vi "ForecastData Test.vi"(8 "error in":errorcluster, 11 "IED Test in":refnum<class "IED Test.lvclass">) -> (0 "error out":errorcluster, 2 "Test Result":T1=enum."Success", 3 "IED Test out":refnum<class "IED Test.lvclass">)   [LabVIEW 2018, in "IED Test Framework.lvlib" / "IED Test.lvclass"]
uses:
  IED Test.lvclass
  C:/Program Files (x86)/National Instruments/LabVIEW 2018/vi.lib/ActorFramework/Actor/Actor.lvclass
  C:/Users/Administrator/Desktop/2018LabVIEW EMS/EMS Generic Actor/EMS Generic/EMS Generic.lvclass
  Controls/Test Result.ctl
  <vilib>/ORNL/CSEISMIC DDS/CSEISMIC DDS Base/Data Types/Controls/DeviceClass Selector.ctl
  ForecastData Actor/ForecastData/ForecastData.lvclass
  C:/Users/Administrator/Desktop/2018LabVIEW EMS/IED Actors/Device DDS Communications Framework/Device DDS Communications/Device DDS Communications.lvclass
  <vilib>/ORNL/CSEISMIC DDS/CSEISMIC DDS Base/CSEISMIC DDS.lvclass/CSEISMIC DDS.ctl
  <vilib>/ORNL/CSEISMIC DDS/CSEISMIC DDS Base/Data Types/Controls/DeviceID.ctl
  <vilib>/ActorFramework/Message Enqueuer/Message Enqueuer.lvclass/Message Enqueuer.ctl
  <vilib>/ORNL/CSEISMIC DDS/CSEISMIC DDS Base/Accessors/Write DDS Reference.vi
  <vilib>/ORNL/CSEISMIC DDS/CSEISMIC DDS Base/Accessors/Read DDS Reference.vi
  <vilib>/ActorFramework/Message Enqueuer/Enqueue.vi
  <vilib>/ORNL/CSEISMIC DDS/DDS Writer/DDS Writer.lvclass
  C:/Program Files (x86)/National Instruments/LabVIEW 2018/vi.lib/ORNL/CSEISMIC DDS/CSEISMIC DDS Base/CSEISMIC DDS.lvclass
  <vilib>/ActorFramework/Stop Msg/Stop Msg.lvclass
  C:/Program Files (x86)/National Instruments/LabVIEW 2018/vi.lib/ActorFramework/Message/Message.lvclass
  <vilib>/ORNL/CSEISMIC DDS/CSEISMIC DDS Base/Error Handler.vi
  <vilib>/ActorFramework/Message Priority Queue/Priority Enqueue.vi
  <vilib>/ORNL/CSEISMIC DDS/CSEISMIC DDS Base/CSEISMIC DDS.lvclass
  Device DDS Communications Framework/Device DDS Communications/Device DDS Communications.lvclass
  <vilib>/ActorFramework/Actor/Actor.lvclass
  EMS Generic Actor/EMS Generic/EMS Generic.lvclass
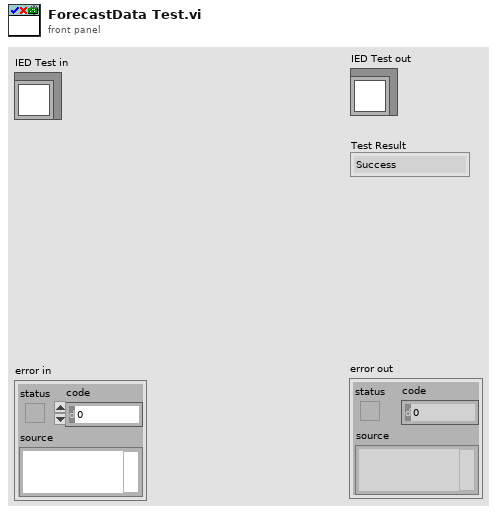
[diagram p1: front panel]
types:
  T1 = typedef "IED Test Framework.lvlib/IED Test.lvclass/Test Result.ctl" = enum16{"Invalid", "Success", "Failure", "Error", "Timeout"}
  T2 = typedef "CSEISMIC DDS.lvlib/CSEISMIC DDS.lvclass/DeviceID.ctl" = string
  T3 = typedef "CSEISMIC DDS.lvlib/CSEISMIC DDS.lvclass/DeviceClass Selector.ctl" = u16
  T4 = typedef "CSEISMIC DDS.lvlib/CSEISMIC DDS.lvclass/ForecastData_Data.ctl" = cluster{"DeviceID":T2, "TargetID":T2, "t0":dbl, "dt":dbl, "Magnitude":dbl[]}
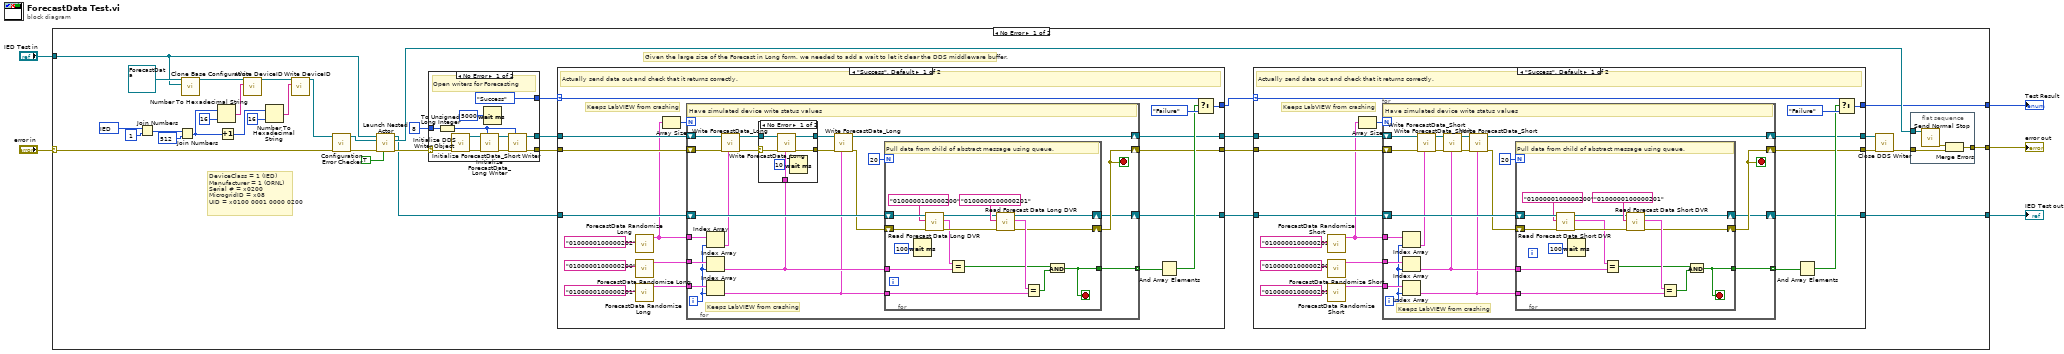
[diagram p0: block diagram]
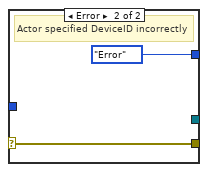
[diagram p5: hidden frame]
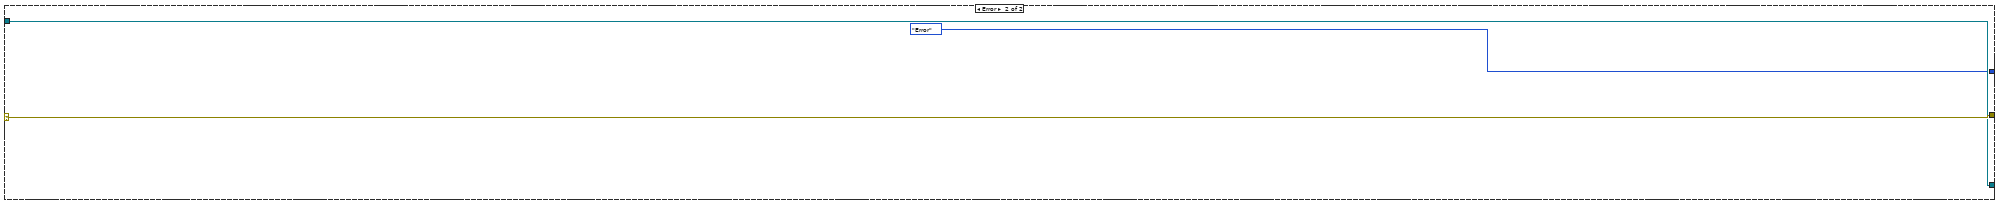
[diagram p6: hidden frame]
diagram:
  n1 = case shown="No Error" "error in" {
    selector: "error in" -> [w37 w185]
    tunnel: [w39 w185] -> w2
    tunnel: [w6 w184] -> w1
    tunnel: "IED Test in" -> [w8 w184]
    tunnel: [w12 Test_Result."Error" ("f")] -> w3
    frame No Error {
      w30 = T3 256 items=["Invalid"=0, "IED"=256, "DER"=512, "Relay"=768, "Meter"=1024, "Load"=1280, "Forecast"=1536, "Price"=1792, "Energy Storage"=513, "PV"=514, "Generator"=515, "Smart Relay"=769, "PCC"=770, "Smart Meter"=1025, "PMU"=1026, "HVAC"=1281] ("DeviceClass")
      # "Given the large size of the Forecast in Long form, we needed to add a wait to let it clear the DDS middleware buffer."
      # "DeviceClass = 1 (IED)\nManufacturer = 1 (ORNL)\nSerial # = x0200\nMicrogridID = x08\nUID = x0100 0001 0000 0200"
      n2 = Join Numbers(hi=w30, lo=u16 1 ("MicrogridID")) -> ((hi.lo)=w27:u32)
      n3 = Join Numbers(hi=w27, lo=u32 512 ("MicrogridID")) -> ((hi.lo)=w32:u64)
      n4 = call-dynamic "Clone Base Configuration.vi"("Source Object"=w8, "Target Object in"=refnum<class "ForecastData.lvclass"> refnum ("ForecastData Actor.lvlib:ForecastData.lvclass")) -> ("Target Object out"=w9:refnum<class "ForecastData.lvclass">)  [unwired: 9 in]
      n5 = Number To Hexadecimal String(1:i16 16 ("width (-)"), 2:w32) -> (0:w25:string)
      n6 = Increment(x=w32) -> (x+1=w34:u64)
      n7 = call-dynamic "Write DeviceID.vi"("DeviceID"=w25, "Device DDS Communications in"=w9) -> ("Device DDS Communications out"=w29:refnum<class "ForecastData.lvclass">)  [unwired: 9 in]
      n8 = Number To Hexadecimal String(1:i16 16 ("width (-)"), 2:w34) -> (0:w35:string)
      n9 = call-dynamic "Write DeviceID.vi"("DeviceID"=w35, "Device DDS Communications in"=w29) -> ("Device DDS Communications out"=w11:refnum<class "ForecastData.lvclass">)  [unwired: 9 in]
      n10 = call "Configuration Error Checker.vi"("error in"=w37, "Device DDS Communications in"=w11) -> ("error out"=w40:errorcluster, "Device DDS Communications out"=w38:refnum<class "ForecastData.lvclass">)  [unwired: 8 in]
      n11 = call <vilib>:"Launch Nested Actor.vi"("Open Actor Core front panel? (F)"=TRUE, "error in (no error)"=w40, "Nested Actor"=w38, "Caller Actor in"=w8) -> ("error out"=w23:errorcluster, "Nested Actor's Enqueuer"=w36:refnum<class "Message Enqueuer.lvclass">, "Caller Actor out"=w16:refnum<class "IED Test.lvclass">)  [unwired: 5 in]
      n12 = case shown="No Error" w23 {
        selector: w23 -> [w178 w182]
        tunnel: [w171 w182] -> w20
        tunnel: u32 8 ("domain id") -> [w180 _]
        tunnel: [Test_Result."Success" ("Test Result in") Test_Result."Error" ("Test Result")] -> w22
        tunnel: [w170 _] -> w21
        frame No Error {
          # "Open writers for Forecasting"
          n13 = To Unsigned Long Integer(number=w180) -> (unsigned 32bit integer=w173:u32)
          n14 = call <vilib>:"Initialize DDS Writer Object.vi"("error in"=w178) -> ("error out"=w177:errorcluster, "DDS Writer out"=w176:refnum<class "DDS Writer.lvclass">)  [unwired: 9 in]
          n15 = call <vilib>:"Initialize ForecastData_Long Writer.vi"("MicrogridID"=w173, "error in"=w177, "DDS Writer in"=w176) -> ("error out"=w174:errorcluster, "DDS Writer out"=w175:refnum<class "DDS Writer.lvclass">)  [unwired: 7 in]
          n16 = Wait (ms)(milliseconds to wait=u32 5000) -> ()  [unwired: 1 out]
          n17 = call <vilib>:"Initialize ForecastData_Short Writer.vi"("MicrogridID"=w173, "error in"=w174, "DDS Writer in"=w175) -> ("error out"=w171:errorcluster, "DDS Writer out"=w170:refnum<class "DDS Writer.lvclass">)  [unwired: 7 in]
        }
        frame Error {
          # "Actor specified DeviceID incorrectly"
        }
      }
      n18 = case shown="\"Success\", Default" w22 {
        selector: w22 -> [w120 w168]
        tunnel: w21 -> [w121 w167]
        tunnel: w16 -> [w115 w166]
        tunnel: w20 -> [w116 w169]
        tunnel: [w118 w168] -> w17
        tunnel: [w114 w169] -> w18
        tunnel: [w112 w167] -> w19
        tunnel: [w104 w166] -> w7
        frame "Success", Default {
          # "Keeps LabVIEW from crashing"
          # "Actually send data out and check that it returns correctly."
          n19 = call "ForecastData Randomize Long.vi"("DeviceID"=T2 "0100000100000202" ("(hi.lo)")) -> ("ForecastData_Long Array out"=w111:T4[])  [unwired: 10 in]
          n20 = call "ForecastData Randomize Long.vi"("DeviceID"=T2 "0100000100000200" ("(hi.lo)")) -> ("ForecastData_Long Array out"=w106:T4[])  [unwired: 10 in]
          n21 = call "ForecastData Randomize Long.vi"("DeviceID"=T2 "0100000100000201" ("(hi.lo)")) -> ("ForecastData_Long Array out"=w107:T4[])  [unwired: 10 in]
          n22 = Array Size(array=w111) -> (size(s)=w113:i32)
          n23 = for {
            N: w113 -> [_]
            shift-right: [w138] -> w112
            shift-left: w121 -> [w141]
            tunnel: w111 -> [w134]
            tunnel: w107 -> [w129]
            tunnel: w106 -> [w130]
            shift-right: [w131] -> w114
            shift-left: w116 -> [w137]
            shift-right: [w125] -> w104
            shift-left: w115 -> [w133]
            tunnel: [w122] -> w105 mode=indexing
            i -> [w127]
            stop <- w131 stop-if-true
            # "Keeps LabVIEW from crashing"
            # "Have simulated device write status values"
            n24 = Index Array(array=w134, index=w127) -> (element=w126:T4)
            n25 = Index Array(array=w130, index=w127) -> (element=w124:T4)
            n26 = Index Array(array=w129, index=w127) -> (element=w123:T4)
            n27 = call <vilib>:"Write ForecastData_Long.vi"("ForecastData"=w126, "error in"=w137, "DDS Writer in"=w141) -> ("error out"=w136:errorcluster, "DDS Writer out"=w140:refnum<class "DDS Writer.lvclass">)  [unwired: 7 in]
            n28 = case shown="No Error" w136 {
              selector: w136 -> [w145 w148]
              tunnel: w140 -> [w147 w149]
              tunnel: [w146 w149] -> w139
              tunnel: [w144 w148] -> w135
              tunnel: w124 -> [w143 _]
              frame No Error {
                n29 = call <vilib>:"Write ForecastData_Long.vi"("ForecastData"=w143, "error in"=w145, "DDS Writer in"=w147) -> ("error out"=w144:errorcluster, "DDS Writer out"=w146:refnum<class "DDS Writer.lvclass">)  [unwired: 7 in]
                n30 = Wait (ms)(milliseconds to wait=u32 10) -> ()  [unwired: 1 out]
              }
              frame Error {
              }
            }
            n31 = call <vilib>:"Write ForecastData_Long.vi"("ForecastData"=w123, "error in"=w135, "DDS Writer in"=w139) -> ("error out"=w132:errorcluster, "DDS Writer out"=w138:refnum<class "DDS Writer.lvclass">)  [unwired: 7 in]
            n32 = for {
              N: 20 -> [_]
              shift-right: [w154] -> w131
              shift-left: w132 -> [w164]
              shift-right: [w155] -> w125
              shift-left: w133 -> [w165]
              tunnel: w124 -> [w159]
              tunnel: w123 -> [w157]
              tunnel: [w151] -> w122
              stop <- w151 stop-if-true
              # "Pull data from child of abstract message using queue."
              n33 = Wait (ms)(milliseconds to wait=u32 100) -> ()  [unwired: 1 out]
              n34 = call "Read Forecast Data Long DVR.vi"("error in"=w164, "DeviceID"=T2 "0100000100000200" ("(hi.lo)"), "EMS Generic in"=w165) -> ("error out"=w160:errorcluster, "ForecastData"=w158:T4, "EMS Generic out"=w161:refnum<class "IED Test.lvclass">)  [unwired: 5 in, 1 out]
              n35 = Equal?(x=w158, y=w159) -> (x = y?=w153:bool)
              n36 = call "Read Forecast Data Long DVR.vi"("error in"=w160, "DeviceID"=T2 "0100000100000201" ("(hi.lo)"), "EMS Generic in"=w161) -> ("error out"=w154:errorcluster, "ForecastData"=w156:T4, "EMS Generic out"=w155:refnum<class "IED Test.lvclass">)  [unwired: 5 in, 1 out]
              n37 = Equal?(x=w156, y=w157) -> (x = y?=w152:bool)
              n38 = And(x=w153, y=w152) -> (x .and. y?=w151:bool)
            }
          }
          n39 = And Array Elements(Boolean array=w105) -> (logical AND=w117:bool)
          n40 = Select(t=w120, s=w117, f=Test_Result."Failure") -> (s? t:f=w118:T1)
        }
        frame "Error" {
        }
      }
      n41 = case shown="\"Success\", Default" w17 {
        selector: w17 -> [w62 w102]
        tunnel: w19 -> [w63 w101]
        tunnel: w7 -> [w57 w100]
        tunnel: w18 -> [w58 w103]
        tunnel: [w60 w102] -> w12
        tunnel: [w56 w103] -> w14
        tunnel: [w54 w101] -> w15
        tunnel: [w47 w100] -> w6
        frame "Success", Default {
          # "Keeps LabVIEW from crashing"
          # "Actually send data out and check that it returns correctly."
          n42 = call "ForecastData Randomize Short.vi"("DeviceID"=T2 "0100000100000202" ("(hi.lo)")) -> ("ForecastData_Short Array out"=w53:T4[])  [unwired: 10 in]
          n43 = call "ForecastData Randomize Short.vi"("DeviceID"=T2 "0100000100000200" ("(hi.lo)")) -> ("ForecastData_Short Array out"=w48:T4[])  [unwired: 10 in]
          n44 = call "ForecastData Randomize Short.vi"("DeviceID"=T2 "0100000100000201" ("(hi.lo)")) -> ("ForecastData_Short Array out"=w49:T4[])  [unwired: 10 in]
          n45 = Array Size(array=w53) -> (size(s)=w55:i32)
          n46 = for {
            N: w55 -> [_]
            shift-right: [w80] -> w54
            shift-left: w63 -> [w83]
            tunnel: w53 -> [w76]
            tunnel: w49 -> [w71]
            tunnel: w48 -> [w72]
            shift-right: [w73] -> w56
            shift-left: w58 -> [w79]
            shift-right: [w67] -> w47
            shift-left: w57 -> [w75]
            tunnel: [w64] -> w46 mode=indexing
            i -> [w69]
            stop <- w73 stop-if-true
            # "Keeps LabVIEW from crashing"
            # "Have simulated device write status values"
            n47 = Index Array(array=w76, index=w69) -> (element=w68:T4)
            n48 = Index Array(array=w72, index=w69) -> (element=w66:T4)
            n49 = Index Array(array=w71, index=w69) -> (element=w65:T4)
            n50 = call <vilib>:"Write ForecastData_Short.vi"("ForecastData"=w68, "error in"=w79, "DDS Writer in"=w83) -> ("error out"=w78:errorcluster, "DDS Writer out"=w82:refnum<class "DDS Writer.lvclass">)  [unwired: 7 in]
            n51 = call <vilib>:"Write ForecastData_Short.vi"("ForecastData"=w66, "error in"=w78, "DDS Writer in"=w82) -> ("error out"=w77:errorcluster, "DDS Writer out"=w81:refnum<class "DDS Writer.lvclass">)  [unwired: 7 in]
            n52 = call <vilib>:"Write ForecastData_Short.vi"("ForecastData"=w65, "error in"=w77, "DDS Writer in"=w81) -> ("error out"=w74:errorcluster, "DDS Writer out"=w80:refnum<class "DDS Writer.lvclass">)  [unwired: 7 in]
            n53 = for {
              N: 20 -> [_]
              shift-right: [w88] -> w73
              shift-left: w74 -> [w99]
              shift-right: [w87] -> w67
              shift-left: w75 -> [w98]
              tunnel: w66 -> [w92]
              tunnel: w65 -> [w91]
              tunnel: [w84] -> w64
              stop <- w84 stop-if-true
              # "Pull data from child of abstract message using queue."
              n54 = call "Read Forecast Data Short DVR.vi"("error in"=w99, "DeviceID"=T2 "0100000100000200" ("(hi.lo)"), "EMS Generic in"=w98) -> ("error out"=w95:errorcluster, "ForecastData"=w90:T4, "EMS Generic out"=w94:refnum<class "IED Test.lvclass">)  [unwired: 5 in, 1 out]
              n55 = Wait (ms)(milliseconds to wait=u32 100) -> ()  [unwired: 1 out]
              n56 = Equal?(x=w90, y=w92) -> (x = y?=w86:bool)
              n57 = call "Read Forecast Data Short DVR.vi"("error in"=w95, "DeviceID"=T2 "0100000100000201" ("(hi.lo)"), "EMS Generic in"=w94) -> ("error out"=w88:errorcluster, "ForecastData"=w89:T4, "EMS Generic out"=w87:refnum<class "IED Test.lvclass">)  [unwired: 5 in, 1 out]
              n58 = Equal?(x=w89, y=w91) -> (x = y?=w85:bool)
              n59 = And(x=w86, y=w85) -> (x .and. y?=w84:bool)
            }
          }
          n60 = And Array Elements(Boolean array=w46) -> (logical AND=w59:bool)
          n61 = Select(t=w62, s=w59, f=Test_Result."Failure") -> (s? t:f=w60:T1)
        }
        frame "Error" {
        }
      }
      n62 = call <vilib>:"Close DDS Writer.vi"("error in"=w14, "DDS Writer in"=w15) -> ("error out"=w13:errorcluster)  [unwired: 9 in]
      n63 = flat-sequence {
        tunnel: w36 -> [w45]
        tunnel: [w43] -> w39
        tunnel: w13 -> [w42]
        frame #0 {
          n64 = call <vilib>:"Send Normal Stop.vi"("Message Enqueuer"=w45) -> ("error out"=w44:errorcluster)  [unwired: 10 in]
          n65 = Merge Errors(w44, w42) -> (w43:errorcluster)
        }
      }
    }
    frame Error {
    }
  }
  "error out" <- w2
  "IED Test out" <- w1
  "Test Result" <- w3
